vi "c REVLib RunDaemon.vi"(8 "error in (no error)":errorcluster) -> (0 "error out":errorcluster, 1 "return type":i32)   [LabVIEW 2026]
uses:
  lib/libREVLibDriver.so
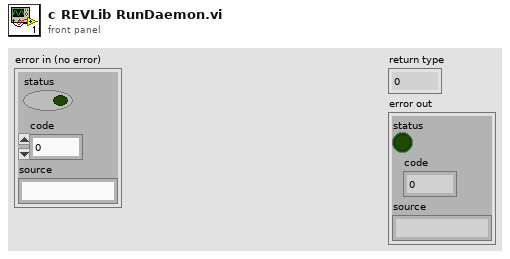
[diagram p1: front panel]
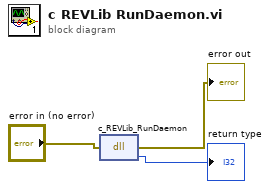
[diagram p0: block diagram]
diagram:
  n1 = dll-call lib="home/systemcore/natinst/lib/libREVLibDriver.so" fn="c_REVLib_RunDaemon"(error in="error in (no error)") -> (error out=→"error out":errorcluster, "return type"=→"return type":i32)  [unwired: 2 in, 1 out]
